vi "SwerveKinematics_ToChassisSpeedsX.vi"(9 "WheelStates":T2[](array[typedef]) {"Angle"."SIN" format="%13.4f"; "Angle"."COS" format="%13.4f"; "Angle"."VALUE" format="%13.4f"}, 11 "in SWERVE_DRIVE_KINEMATICS":T4 {"PrevCoR"."Y" format="%14.3f"; "PrevCoR"."X" format="%14.3f"; "Modules"."Y" format="%14.3f"; "Modules"."X" format="%14.3f"}) -> (1 "Chassis Speed":T1 {"vOmega" format="%10.3f"; "vY" format="%10.3f"; "vX" format="%10.3f"})   [LabVIEW 2019, in "Trajectory_Library.lvlib"]
doc: "Performs forward kinematics to return the resulting chassis state from the given module states. This method is often used for odometry -- determining the robot's position on the field using data from the real-world speed and angle of each module on the robot.\n\nParameters: \n - in Swerve Drive Kinematics - Swerve drive kinematics data structure\n - wheelStates - The state of the modules (as a SwerveModuleState type) as measured from respective encoders and gyros. The order of the swerve module states should be same as passed into the constructor of this class.\n\nReturns:\n - The resulting chassis speed."
uses:
  Trajectory_Library.lvlib
  SWERVE_DRIVE_KINEMATICS.ctl
  TRANSLATION2D.ctl
  SWERVE_DRIVE_MODULE_STATE.ctl
  ROTATION2D.ctl
  CHASSIS_SPEEDS.ctl
  <vilib>/Analysis/Matrix/Numeric/Multiply/Multiply - RM,RM.vi
  <vilib>/Analysis/Matrix/NI_Matrix.lvlib
  <vilib>/Analysis/Matrix/Datatypes/RealMatrix.ctl
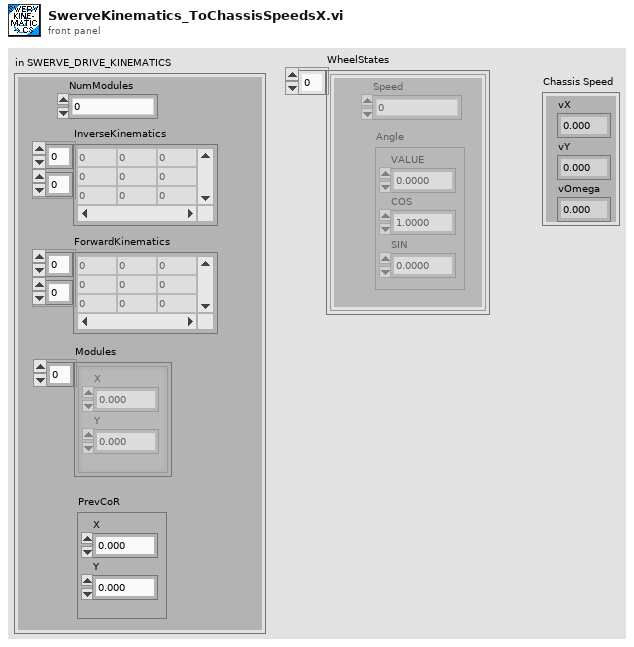
[diagram p1: front panel]
types:
  T1 = typedef "Trajectory_Library.lvlib/CHASSIS_SPEEDS.ctl" = cluster{"vX":dbl, "vY":dbl, "vOmega":dbl}
  T2 = typedef "Trajectory_Library.lvlib/SWERVE_DRIVE_MODULE_STATE.ctl" = cluster{"Speed":dbl, "Angle":T3}
  T3 = typedef "Trajectory_Library.lvlib/ROTATION2D.ctl" = cluster{"VALUE":dbl, "COS":dbl, "SIN":dbl}
  T4 = typedef "Trajectory_Library.lvlib/SWERVE_DRIVE_KINEMATICS.ctl" = cluster{"NumModules":i32, "InverseKinematics":T5, "ForwardKinematics":T5, "Modules":T6[], "PrevCoR":T6}
  T5 = typedef "NI_Matrix.lvlib/RealMatrix.ctl" = dbl[][]
  T6 = typedef "Trajectory_Library.lvlib/TRANSLATION2D.ctl" = cluster{"X":dbl, "Y":dbl}
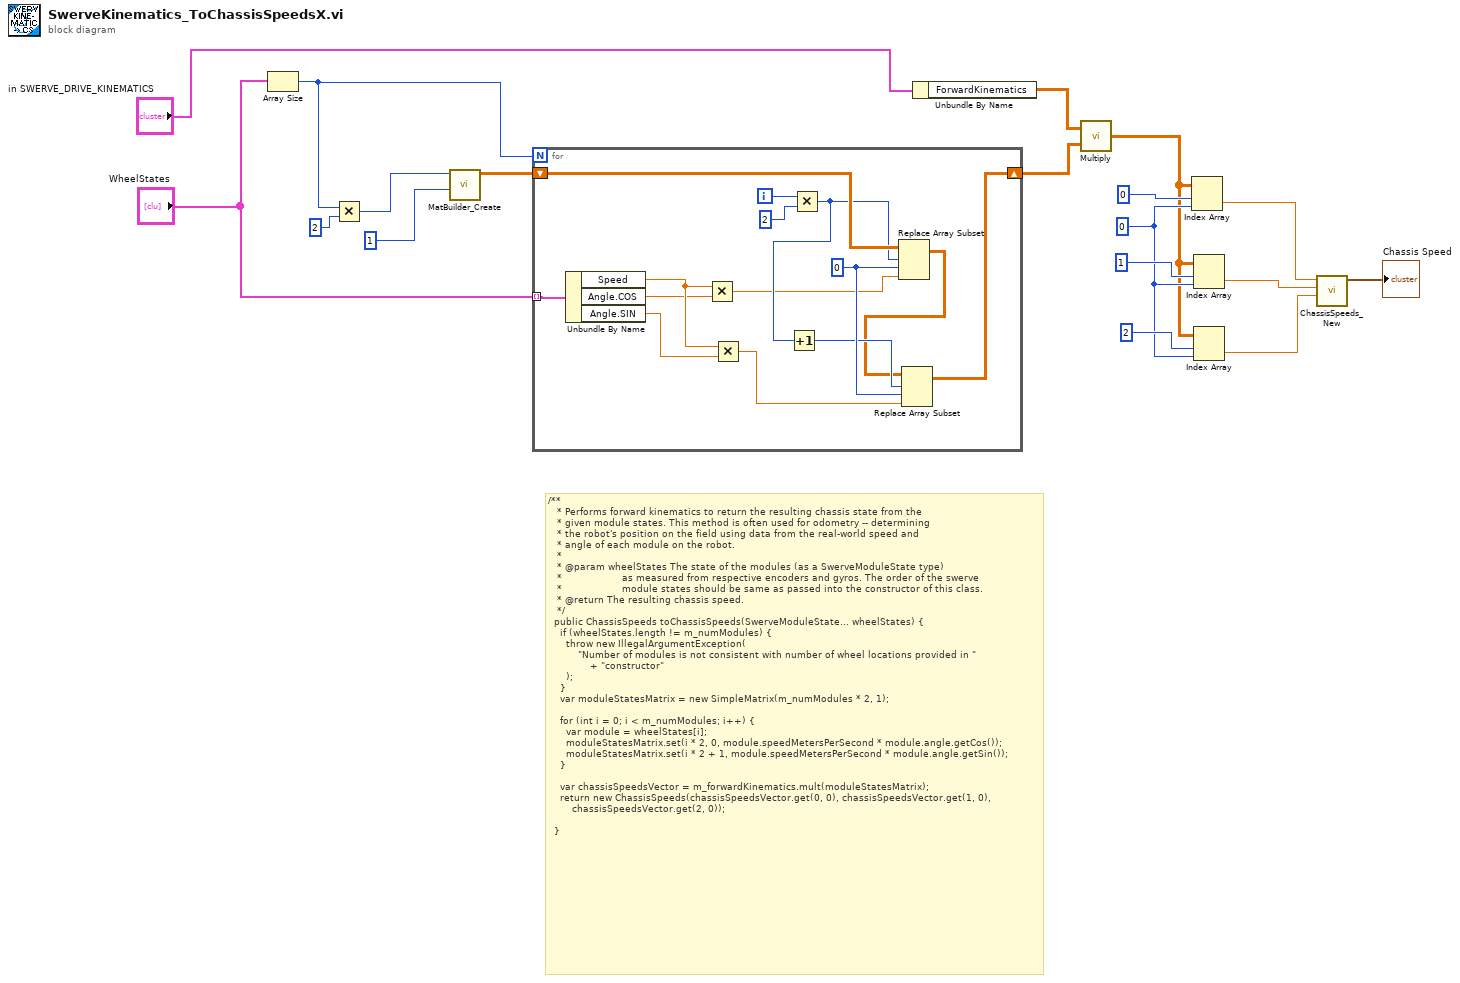
[diagram p0: block diagram]
diagram:
  w9 = 0 ("index (col)")
  # "/**\n   * Performs forward kinematics to return the resulting chassis state from the\n   * given module states. This method is often used for odometry -- determining\n   * the robot's position on the field using data from the real-world speed and\n   * angle of each module on the robot.\n   *\n   * @param wheelStates The state of the modules (as a SwerveModuleState type)\n   *                    as measured from respective encoders and gyros. The order of the swerve\n   *                    module states should be same as passed into the constructor of this class.\n   * @return The resulting chassis speed.\n   */\n  public ChassisSpeeds toChassisSpeeds(SwerveModuleState... wheelStates) {\n    if (wheelStates.length != m_numModules) {\n      throw new IllegalArgumentException(\n          \"Number of modules is not consistent with number of wheel locations provided in \"\n              + \"constructor\"\n      );\n    }\n    var moduleStatesMatrix = new SimpleMatrix(m_numModules * 2, 1);\n\n    for (int i = 0; i < m_numModules; i++) {\n      var module = wheelStates[i];\n      moduleStatesMatrix.set(i * 2, 0, module.speedMetersPerSecond * module.angle.getCos());\n      moduleStatesMatrix.set(i * 2 + 1, module.speedMetersPerSecond * module.angle.getSin());\n    }\n\n    var chassisSpeedsVector = m_forwardKinematics.mult(moduleStatesMatrix);\n    return new ChassisSpeeds(chassisSpeedsVector.get(0, 0), chassisSpeedsVector.get(1, 0),\n        chassisSpeedsVector.get(2, 0));\n\n  }"
  n1 = Array Size(array="WheelStates") -> (size(s)=w17:i32)
  n2 = Multiply(x=w17, y=2) -> (x*y=w3:i32)
  n3 = call "MatBuilder_Create.vi"("Columns"=1 ("number of columns"), "Rows"=w3) -> ("output matrix"=w1:T5)  [unwired: 9 in]
  n4 = for {
    N: w17 -> [_]
    shift-right: [w24] -> w14
    shift-left: w1 -> [w32]
    tunnel: "WheelStates" -> [w26] mode=indexing
    i -> [w30]
    w31 = 0 ("disabled index (col)")
    n5 = Unbundle By Name(w26) -> ("Speed"=w23:dbl, "Angle.COS"=w22:dbl, "Angle.SIN"=w21:dbl)
    n6 = Multiply(x=w23, y=w22) -> (x*y=w20:dbl)
    n7 = Multiply(x=w23, y=w21) -> (x*y=w19:dbl)
    n8 = Multiply(x=w30, y=2) -> (x*y=w28:i32)
    n9 = Increment(x=w28) -> (x+1=w27:i32)
    n10 = Replace Array Subset(array=w32, new element=w20, index (row)=w28, index (col)=w31) -> (w25:T5)
    n11 = Replace Array Subset(array=w25, new element=w19, index (row)=w27, index (col)=w31) -> (w24:T5)
  }
  n12 = Unbundle By Name("in SWERVE_DRIVE_KINEMATICS") -> ("ForwardKinematics"=w15:T5)
  n13 = call-poly <vilib>:"Multiply.vi"("Real Matrix B"=w14, "Real Matrix A"=w15) -> ("A * B"=w8:T5)
  n14 = Index Array(array=w8, index (row)=0, index (col)=w9) -> (element=w7:dbl)
  n15 = Index Array(array=w8, index (row)=1, index (col)=w9) -> (element=w6:dbl)
  n16 = Index Array(array=w8, index (row)=2, index (col)=w9) -> (element=w5:dbl)
  n17 = call "ChassisSpeeds_New.vi"("vAngular"=w5, "vY"=w6, "vX"=w7) -> ("CHASSIS"=→"Chassis Speed":T1)  [unwired: 8 in]
